vi "SolvePuzzle.vi"(8 "error in (no error)":errorcluster, 11 "Puzzle in":refnum<class "Graph.lvclass">) -> (0 "error out":errorcluster, 2 "Solution":i32[][](array[numeric]), 3 "Puzzle out":refnum<class "Graph.lvclass">)   [LabVIEW 2009, in "SudokuBoard.lvclass"]
uses:
  SudokuBoard.lvclass
  Graph/Graph.lvclass
  SudukuState/SudokuState.lvclass
  Graph/SearchMethod.ctl
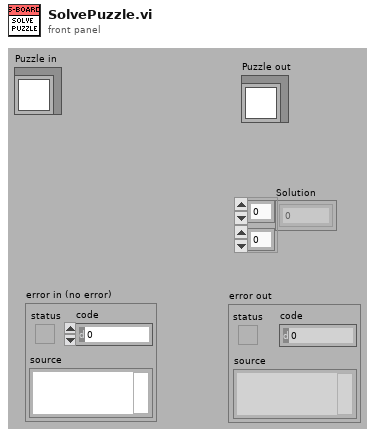
[diagram p1: front panel]
types:
  T1 = typedef "Graph.lvclass/SearchMethod.ctl" = enum16{"Breadth (First)", "Depth (First)", "Best First", "Breadth (Best)", "Depth (Best)"}
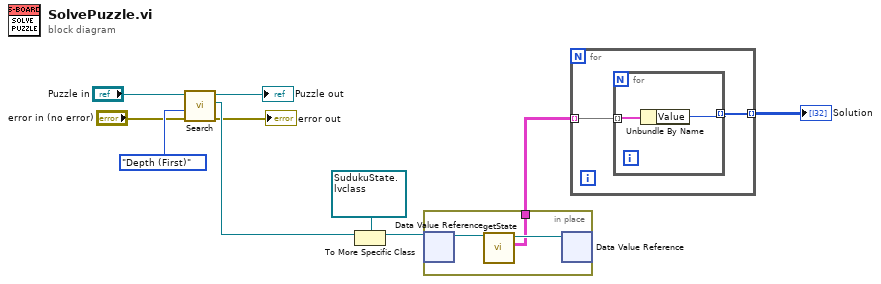
[diagram p0: block diagram]
diagram:
  n1 = call "Search.vi"("error in (no error)"="error in (no error)", "SearchMethod"=SearchMethod."Depth (First)", "Graph in"="Puzzle in") -> ("error out"=→"error out":errorcluster, "Node"=w8:refnum<data-value>, "Graph out"=→"Puzzle out":refnum<class "Graph.lvclass">)  [unwired: 5 in, 1 out]
  n2 = To More Specific Class(target class=refnum<data-value> refnum ("data value reference"), reference=w8) -> (specific class reference=w10:refnum<data-value>)  [unwired: 1 in, 1 out]
  n3 = in-place {
    in-place-border: [w11] -> w6
    n4 = in-place-dvr #1(w10) -> (w13:refnum<class "SudokuState.lvclass">)  [unwired: 1 out]
    n5 = call "getState.vi"("SudukuState in"=w13) -> ("State"=w11:cluster{"Value":i32, "Options":i32[]}[][], "SudukuState out"=w12:refnum<class "SudokuState.lvclass">)  [unwired: 8 in, 1 out]
    n6 = in-place-dvr #1(w12) -> ()  [unwired: 2 out]
  }
  n7 = for {
    tunnel: w6 -> [w15] mode=indexing
    tunnel: [w14] -> w5 mode=indexing
    n8 = for {
      tunnel: w15 -> [w17] mode=indexing
      tunnel: [w16] -> w14 mode=indexing
      n9 = Unbundle By Name(w17) -> ("Value"=w16:i32)
    }
  }
  "Solution" <- w5
